vi "SetErrorLogFile.vi"(2 "ErrorLogFile":refnum<class "ErrorLogFile.lvclass">, 5 "Error In":errorcluster) -> (19 "Error Out":errorcluster)   [LabVIEW 2018, in "Error handler.lvclass"]
uses:
  Error handler.lvclass
  ErrorLogFile_class/ErrorLogFile.lvclass
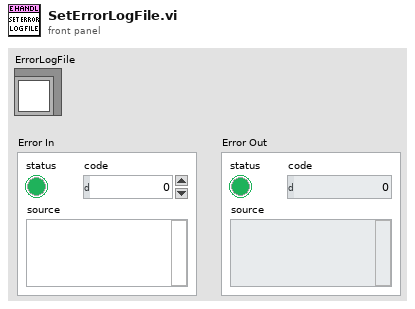
[diagram p1: front panel]
types:
  T1 = typedef "Error handler.lvclass/ObjectAttributes.ctl" = cluster{"ErrorBroadcastEvent":refnum<user-event>, "LoadFPOnError":bool, "ErrorLogFile":refnum<class "ErrorLogFile.lvclass">, "Testing":bool, "Name":string}
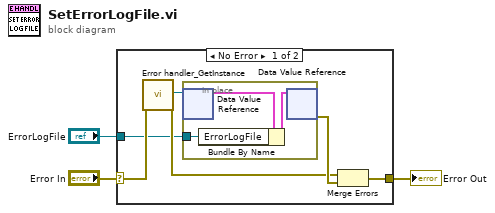
[diagram p0: block diagram]
diagram:
  n1 = case shown="No Error" "Error In" {
    selector: "Error In" -> [w9 w13]
    tunnel: [w6 w13] -> w2
    tunnel: "ErrorLogFile" -> [w4 _]
    frame No Error {
      n2 = call "Error handler_GetInstance.vi"("error in"=w9) -> ("DVRRefOut"=w5:refnum<data-value>, "error out"=w7:errorcluster)  [unwired: 14 in, 3 out]
      n3 = in-place {
        in-place-border: w4 -> [w12]
        n4 = in-place-dvr #1(w5) -> (w11:T1)  [unwired: 1 out]
        n5 = Bundle By Name(cluster=w11, "ErrorLogFile"=w12) -> (w10:T1)
        n6 = in-place-dvr #1(w10) -> (w8:errorcluster)  [unwired: 1 out]
      }
      n7 = Merge Errors(w7, w8) -> (w6:errorcluster)
    }
    frame Error {
    }
  }
  "Error Out" <- w2
